vi "TCL Get Current Fragments - NeventNfrag.vi"(3 "error in (no error)":errorcluster, 4 "fragments":string[](array[string]), 5 "event numbers":i32[](array[numeric])) -> (0 "error out":errorcluster, 1 "values":string[][](array[string]), 2 "fragments out":string[](array[string]))   [LabVIEW 2010]
uses:
  TCL Global.vi
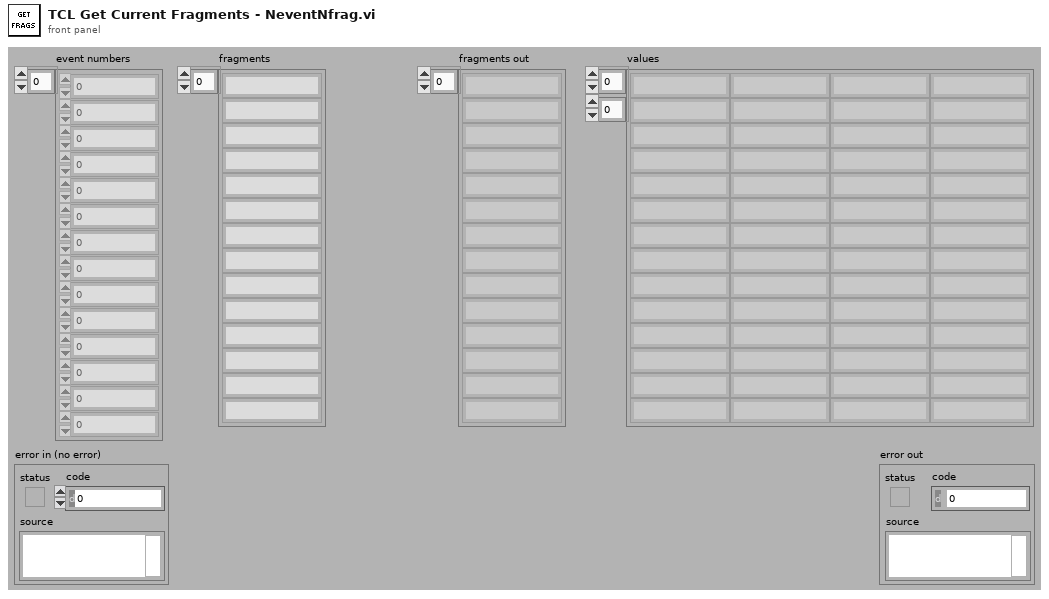
[diagram p1: front panel]
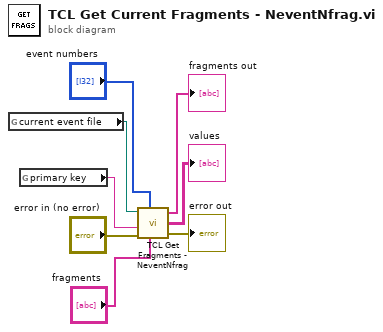
[diagram p0: block diagram]
diagram:
  n1 = global read "TCL Global.vi" "current event file"() -> (w2:path)
  n2 = global read "TCL Global.vi" "primary key"() -> (w1:string)
  n3 = call "TCL Get Fragments - NeventNfrag.vi"("event file"=w2, "event numbers"="event numbers", "primary key"=w1, "fragments"="fragments", "error in (no error)"="error in (no error)") -> ("fragments out"=→"fragments out":string[], "values"=→"values":string[][], "error out"=→"error out":errorcluster)  [unwired: 1 in]
